vi "SetEncScanSpan.vi"(8 "错误输入（无错误）":errorcluster, 10 "编码器序号":i32, 11 "滤波器系数":u32) -> (0 "错误输出":errorcluster)   [LabVIEW 2014]
uses:
  X86Dll/ZXUTConfigMgr.dll
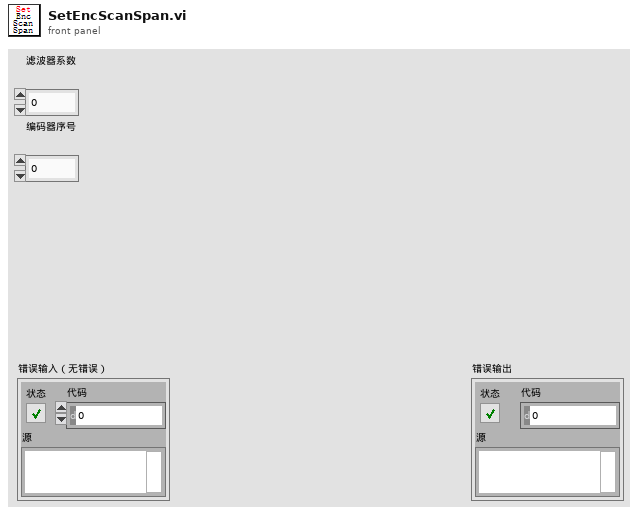
[diagram p1: front panel]
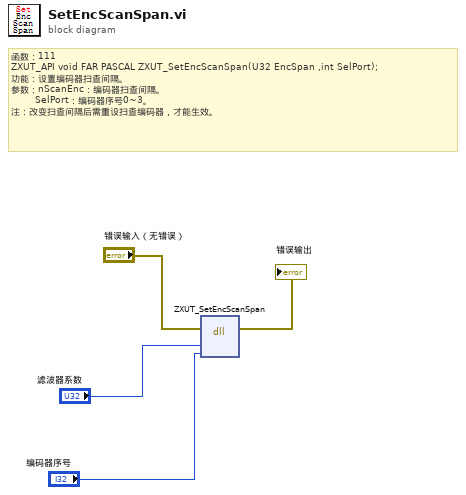
[diagram p0: block diagram]
diagram:
  # "函数：111\nZXUT_API void\tFAR PASCAL ZXUT_SetEncScanSpan(U32 EncSpan ,int SelPort);\n功能：设置编码器扫查间隔。\n参数：nScanEnc：编码器扫查间隔。\n        SelPort：编码器序号0~3。\n注：改变扫查间隔后需重设扫查编码器，才能生效。"
  n1 = dll-call lib="D:/Software/Utrasonic on-line monitoring/X86Dll/ZXUTConfigMgr.dll" fn="ZXUT_SetEncScanSpan"(error in="错误输入（无错误）", "EncSpan"="滤波器系数", "SelPort"="编码器序号") -> (error out=→"错误输出":errorcluster)  [unwired: 5 in, 1 out]
